vi "RT Main FPGA Test.vi"() -> ()   [LabVIEW 2014]
uses:
  controls/FPGA VI Reference.ctl
  controls/Master Configuration.ctl
  controls/EPICS Configuration.ctl
  Globals/Global - All RT Loop Stop.vi
  Globals/Global - Monitoring Variables.vi
  Globals/Global - Configuration Options.vi
  support/Message Queue/Message Queue.lvlib
  <vilib>/nisyscfg/nisyscfg.lvlib
panel:
  in  "Index":u32
  in  "Message":string
  in  "Send":bool
  in  "stop":bool
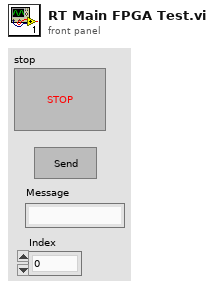
[diagram p1: front panel]
types:
  T1 = typedef "FPGA VI Reference.ctl" = refnum<k20>
  T2 = typedef "Master Configuration.ctl" = cluster{"Thresholds":dbl[], "Epics Configuration":T3, "Epics Configuration File":string, "Number of Channels":dbl}
  T3 = typedef "EPICS Configuration.ctl" = cluster{"Data rate":u32, "Input active":bool[], "# Samples Post Trig":u32, "Armed":bool}
  T4 = typedef "Message Queue.lvlib/All Real-Time Message Queues.ctl" = cluster{"Message Handler":refnum<queue>, "FPGA Subsystem":refnum<queue>}
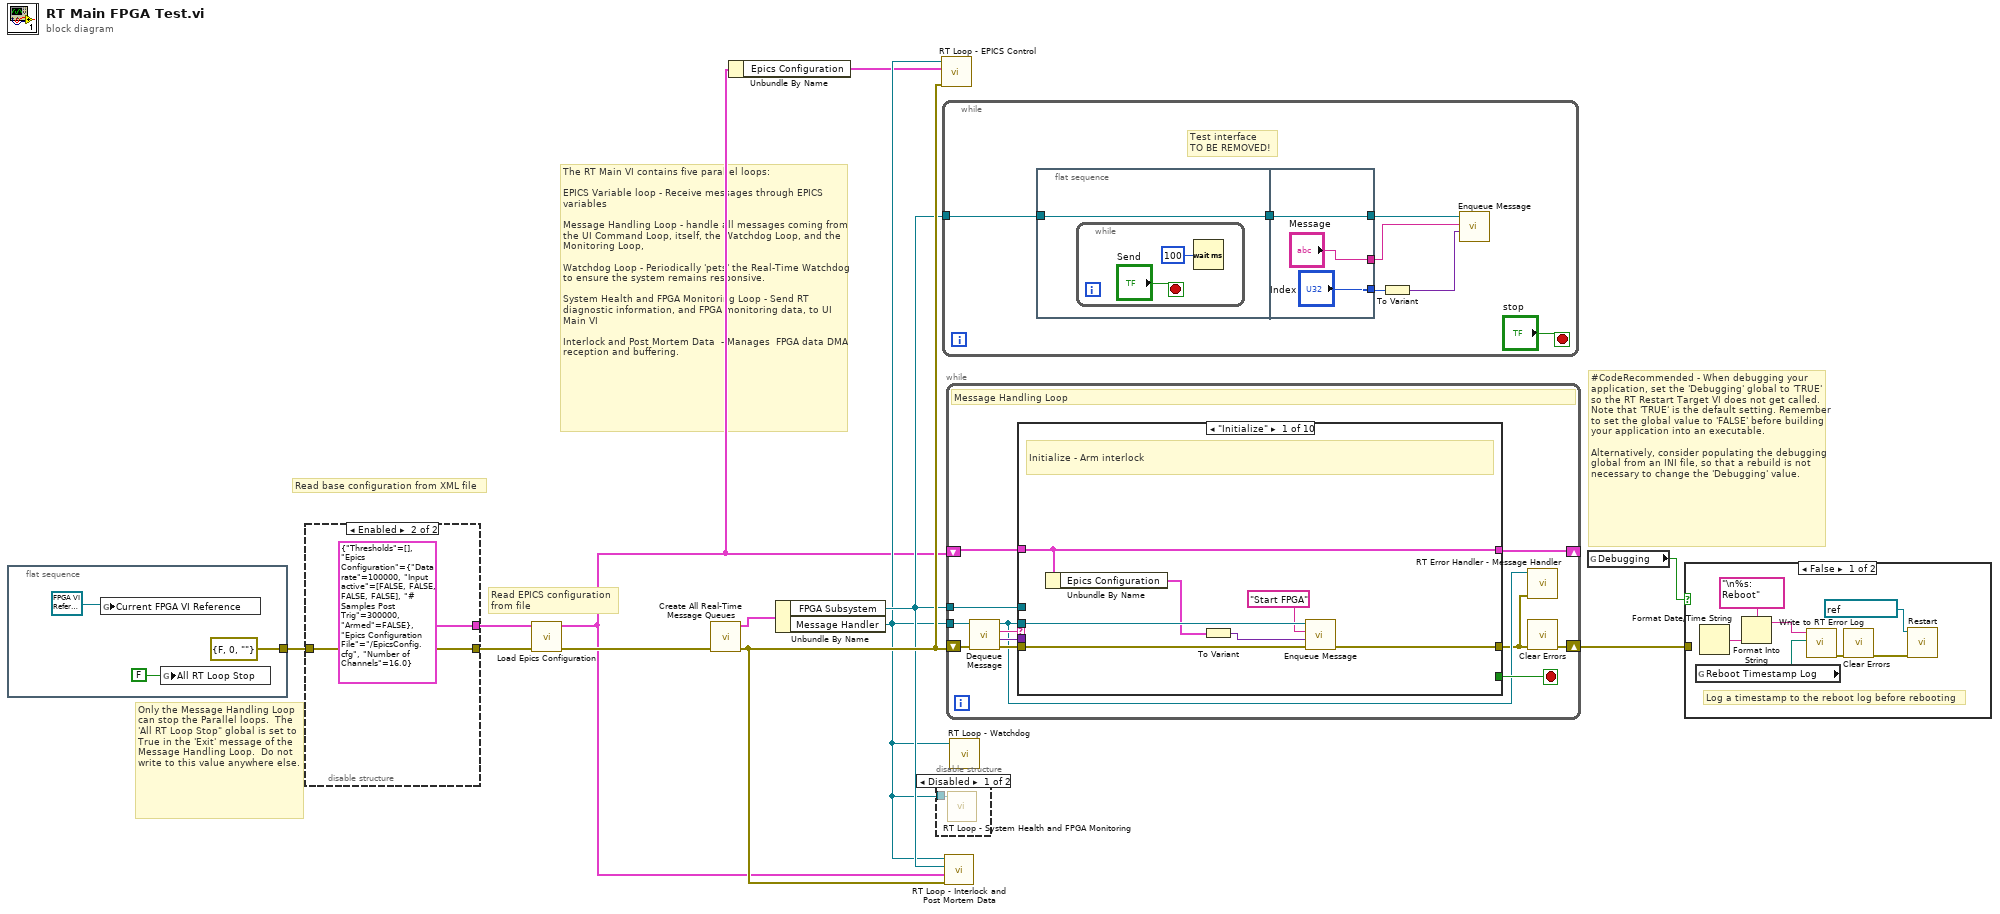
[diagram p0: block diagram]
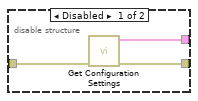
[diagram p3: hidden frame]
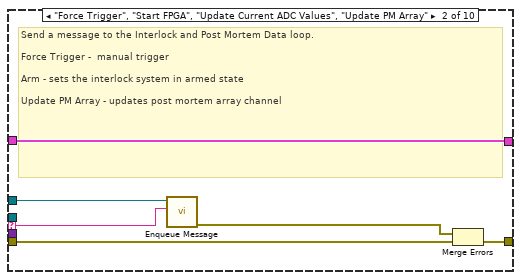
[diagram p5: hidden frame]
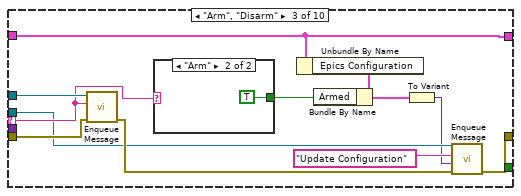
[diagram p6: hidden frame]
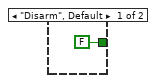
[diagram p7: hidden frame]
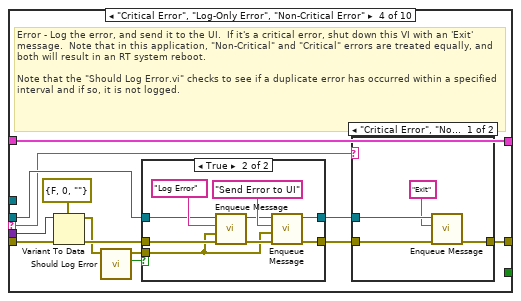
[diagram p8: hidden frame]
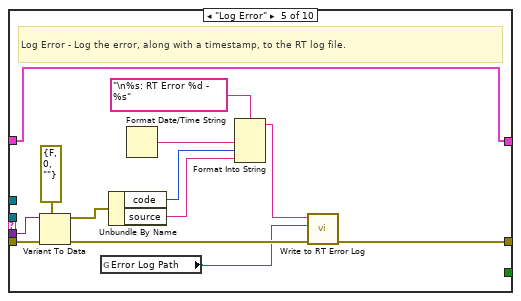
[diagram p11: hidden frame]
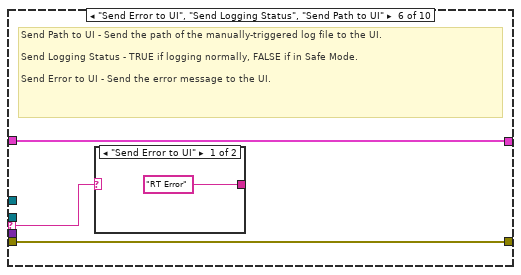
[diagram p12: hidden frame]
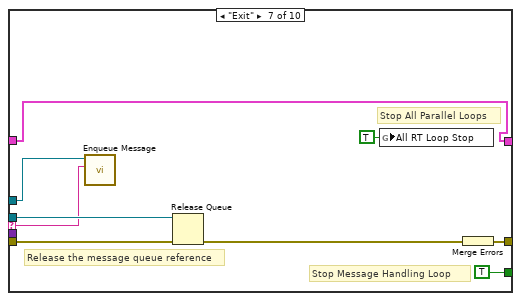
[diagram p14: hidden frame]
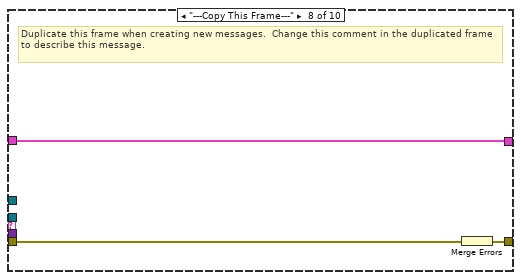
[diagram p15: hidden frame]
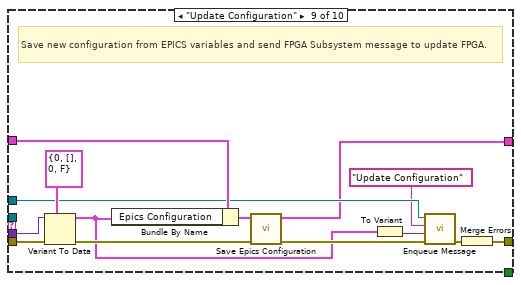
[diagram p16: hidden frame]
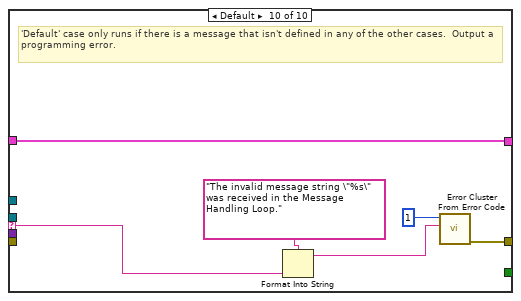
[diagram p17: hidden frame]
diagram:
  # "Read EPICS configuration\nfrom file"
  # "Read base configuration from XML file"
  # "#CodeRecommended - When debugging your application, set the 'Debugging' global to 'TRUE' so the RT Restart Target VI does not get called.  Note that 'TRUE' is the default setting. Remember to set the global value to 'FALSE' before building your application into an executable.\n\nAlternatively, consider populating the debugging global from an INI file, so that a rebuild is not necessary to change the 'Debugging' value."
  # "The RT Main VI contains five parallel loops:\n\nEPICS Variable loop - Receive messages through EPICS variables\n\nMessage Handling Loop - handle all messages coming from the UI Command Loop, itself, the Watchdog Loop, and the Monitoring Loop, \n\nWatchdog Loop - Periodically 'pets' the Real-Time Watchdog to ensure the system remains responsive.\n\nSystem Health and FPGA Monitoring Loop - Send RT diagnostic information, and FPGA monitoring data, to UI Main VI\n\nInterlock and Post Mortem Data  - Manages  FPGA data DMA reception and buffering."
  # "Only the Message Handling Loop can stop the Parallel loops.  The 'All RT Loop Stop\" global is set to True in the 'Exit' message of the Message Handling Loop.  Do not write to this value anywhere else."
  n1 = flat-sequence {
    tunnel: [errorcluster {"status"=FALSE, "code"=0, "source"=""} ("error constant")] -> w12
    frame #0 {
      n2 = global write "Global - Monitoring Variables.vi" "Current FPGA VI Reference"(T1 refnum ("Current FPGA VI Reference")) -> ()
      n3 = global write "Global - All RT Loop Stop.vi" "All RT Loop Stop"(FALSE) -> ()
    }
  }
  n4 = disable-structure shown="Enabled" {
    disable-tunnel: w12 -> [w18 w19]
    disable-tunnel: [w17 w19] -> w6
    disable-tunnel: [w16 T2 {"Thresholds"=[], "Epics Configuration"={"Data rate"=100000, "Input active"=[FALSE, FALSE, FALSE, FALSE], "# Samples Post Trig"=300000, "Armed"=FALSE}, "Epics Configuration File"="/EpicsConfig.cfg", "Number of Channels"=16.0} ("Acquisition and Logging Configuration")] -> w4
    frame Disabled {
      n5 = call "Get Configuration Settings.vi"("error in (no error)"=w18) -> ("error out"=w17:errorcluster, "Acquisition and Logging Configuration"=w16:T2)  [unwired: 9 in]
    }
    frame Enabled {
    }
  }
  n6 = call "Load Epics Configuration.vi"("error in (no error)"=w6, "Master Configuration in"=w4) -> ("error out"=w5:errorcluster, "Master Configuration out"=w2:T2)  [unwired: 8 in]
  n7 = call "Create All Real-Time Message Queues.vi"("error in (no error)"=w5) -> ("error out"=w8:errorcluster, "Message Queues out"=w9:T4)  [unwired: 9 in]
  n8 = Unbundle By Name(w2) -> ("Epics Configuration"=w1:T3)
  n9 = Unbundle By Name(w9) -> ("FPGA Subsystem"=w7:refnum<queue>, "Message Handler"=w3:refnum<queue>)
  n10 = disable-structure shown="Disabled" {
    disable-tunnel: w3 -> [w21 _]
    frame Disabled {
      n11 = call "RT Loop - System Health and FPGA Monitoring.vi"("Message Queue"=w21) -> ()  [unwired: 11 in]
    }
    frame Enabled {
    }
  }
  n12 = call "RT Loop - EPICS Control.vi"("Error"=w8, "Epics Configuration"=w1, "Message Handler"=w3) -> ()  [unwired: 9 in]
  n13 = while {
    tunnel: w7 -> [w27]
    stop <- "stop" stop-if-true
    # "Test interface\nTO BE REMOVED!"
    n14 = flat-sequence {
      tunnel: w27 -> [w29]
      tunnel: [w29] -> w25
      tunnel: [w34] -> w26
      tunnel: w25 -> [w34]
      tunnel: ["Message"] -> w24
      tunnel: ["Index"] -> w23
      frame #0 {
        n15 = while {
          stop <- "Send" stop-if-true
          n16 = Wait (ms)(milliseconds to wait=u32 100) -> ()  [unwired: 1 out]
        }
      }
      frame #1 {
      }
    }
    n17 = To Variant(anything=w23) -> (Variant=w22:variant)
    n18 = call "Enqueue Message.vi"("Message Data"=w22, "Message"=w24, "Message Queue"=w26) -> ()  [unwired: 7 in, 2 out]
  }
  n19 = call "RT Loop - Interlock and Post Mortem Data.vi"("error in (no error)"=w8, "Master Configuration"=w2, "FPGA Subsystem"=w7, "Message Handler"=w3) -> ()  [unwired: 8 in]
  n20 = while {
    tunnel: w3 -> [w41]
    shift-right: [w39] -> w11
    shift-left: w8 -> [w45]
    tunnel: w7 -> [w37]
    shift-right: [w35] -> _
    shift-left: w2 -> [w36]
    stop <- w46 stop-if-true
    # "Message Handling Loop"
    n21 = call "Dequeue Message.vi"("error in (no error)"=w45, "Message Queue"=w41) -> ("error out"=w44:errorcluster, "Message Data"=w42:variant, "Message"=w43:string, "dup Message Queue"=w40:refnum<queue>)  [unwired: 6 in]
    n22 = case "Message Cases" shown="\"Initialize\"" w43 {
      selector: w43 -> [_ w57 w70 w80 _ w117 w122 _ _ w151]
      tunnel: w40 -> [w53 _ w66 w81 _ _ w129 _ _ _]
      tunnel: w44 -> [w52 w59 w68 w83 w115 w118 w125 w132 w146 _]
      tunnel: [w51 w56 w65 w86 w106 w118 w126 w131 w145 w149] -> w38
      tunnel: [_ _ _ _ _ _ TRUE _ _ _] -> w46
      tunnel: w42 -> [_ _ _ w75 w114 _ _ _ w144 _]
      tunnel: w37 -> [_ w58 w71 _ _ _ w123 _ w138 _]
      tunnel: w36 -> [w49 w54 w61 w74 w103 w116 w121 w130 w142 w147]
      tunnel: [w49 w54 w61 w74 w103 w116 w121 w130 w134 w147] -> w35
      frame "Initialize" {
        # "Initialize - Arm interlock"
        n23 = Unbundle By Name(w49) -> ("Epics Configuration"=w48:T3)
        n24 = To Variant(anything=w48) -> (Variant=w47:variant)
        n25 = call "Enqueue Message.vi"("error in (no error)"=w52, "Message Data"=w47, "Message"="Start FPGA", "Message Queue"=w53) -> ("error out"=w51:errorcluster)  [unwired: 6 in, 1 out]
      }
      frame "Force Trigger", "Start FPGA", "Update Current ADC Values", "Update PM Array" {
        # "Send a message to the Interlock and Post Mortem Data loop.\n\nForce Trigger -  manual trigger\n\nArm - sets the interlock system in armed state\n\nUpdate PM Array - updates post mortem array channel"
        n26 = call "Enqueue Message.vi"("Message"=w57, "Message Queue"=w58) -> ("error out"=w55:errorcluster)  [unwired: 8 in, 1 out]
        n27 = Merge Errors(w55, w59) -> (w56:errorcluster)
      }
      frame "Arm", "Disarm" {
        n28 = call "Enqueue Message.vi"("error in (no error)"=w68, "Message"=w70, "Message Queue"=w71) -> ("error out"=w67:errorcluster)  [unwired: 7 in, 1 out]
        n29 = case shown="\"Arm\"" w70 {
          tunnel: [FALSE ("Armed") TRUE ("Armed")] -> w69
          frame "Disarm", Default {
          }
          frame "Arm" {
          }
        }
        n30 = Unbundle By Name(w61) -> ("Epics Configuration"=w60:T3)
        n31 = Bundle By Name(cluster=w60, "Armed"=w69) -> (w63:T3)
        n32 = To Variant(anything=w63) -> (Variant=w62:variant)
        n33 = call "Enqueue Message.vi"("error in (no error)"=w67, "Message Data"=w62, "Message"="Update Configuration", "Message Queue"=w66) -> ("error out"=w65:errorcluster)  [unwired: 6 in, 1 out]
      }
      frame "Critical Error", "Log-Only Error", "Non-Critical Error" {
        # "Error - Log the error, and send it to the UI.  If it's a critical error, shut down this VI with an 'Exit' message.  Note that in this application, \"Non-Critical\" and \"Critical\" errors are treated equally, and both will result in an RT system reboot.\n\nNote that the \"Should Log Error.vi\" checks to see if a duplicate error has occurred within a specified interval and if so, it is not logged."
        n34 = Variant To Data(error in=w83, type=errorcluster {"status"=FALSE, "code"=0, "source"=""} ("error out"), Variant=w75) -> (data=w78:errorcluster, error out=w84:errorcluster)
        n35 = call "Should Log Error.vi"("error to report"=w78) -> ("Should Log Error?"=w76:bool, "dup error to report"=w77:errorcluster)  [unwired: 9 in]
        n36 = case shown="True" w76 {
          tunnel: [w88 w95] -> w82
          tunnel: [w87 w94] -> w79
          tunnel: w81 -> [w87 w93]
          tunnel: w84 -> [w88 w90]
          tunnel: w77 -> [_ w89]
          frame False {
          }
          frame True {
            n37 = call "Enqueue Message.vi"("error in (no error)"=w90, "Message Data"=w89, "Message"="Log Error", "Message Queue"=w93) -> ("error out"=w91:errorcluster, "dup Message Queue"=w92:refnum<queue>)  [unwired: 6 in]
            n38 = call "Enqueue Message.vi"("error in (no error)"=w91, "Message Data"=w89, "Message"="Send Error to UI", "Message Queue"=w92) -> ("error out"=w95:errorcluster, "dup Message Queue"=w94:refnum<queue>)  [unwired: 6 in]
          }
        }
        n39 = case shown="\"Critical Error\", \"Non-Critical Error\"" w80 {
          tunnel: w82 -> [w101 w102]
          tunnel: w79 -> [w99 _]
          tunnel: [w100 w102] -> w86
          frame "Critical Error", "Non-Critical Error" {
            n40 = call "Enqueue Message.vi"("error in (no error)"=w101, "Message"="Exit", "Message Queue"=w99) -> ("error out"=w100:errorcluster)  [unwired: 7 in, 1 out]
          }
          frame Default {
          }
        }
      }
      frame "Log Error" {
        # "Log Error - Log the error, along with a timestamp, to the RT log file."
        n41 = Variant To Data(error in=w115, type=errorcluster {"status"=FALSE, "code"=0, "source"=""} ("error constant"), Variant=w114) -> (data=w109:errorcluster, error out=w112:errorcluster)
        n42 = global read "Global - Configuration Options.vi" "Error Log Path"() -> (w104:path)
        n43 = Unbundle By Name(w109) -> ("code"=w108:i32, "source"=w107:string)
        n44 = Format Date/Time String() -> (date/time string=w110:string)  [unwired: 3 in]
        n45 = Format Into String(format string="\n%s: RT Error %d - %s", w110, w108, w107) -> (resulting string=w105:string)  [unwired: 2 in, 1 out]
        n46 = call "Write to RT Error Log.vi"("error in (no error)"=w112, "Error Log Path"=w104, "Log Entry"=w105) -> ("error out"=w106:errorcluster)  [unwired: 8 in]
      }
      frame "Send Error to UI", "Send Logging Status", "Send Path to UI" {
        # "Send Path to UI - Send the path of the manually-triggered log file to the UI.\n\nSend Logging Status - TRUE if logging normally, FALSE if in Safe Mode.\n\nSend Error to UI - Send the error message to the UI."
        n47 = case shown="\"Send Error to UI\"" w117 {
          selector: w117 -> [_ w120]
          tunnel: ["RT Error" ("Message") w120] -> _
          frame "Send Error to UI" {
          }
          frame Default {
          }
        }
      }
      frame "Exit" {
        # "Stop Message Handling Loop"
        # "Stop All Parallel Loops"
        # "Release the message queue reference"
        n48 = call "Enqueue Message.vi"("Message"=w122, "Message Queue"=w123) -> ()  [unwired: 8 in, 2 out]
        n49 = Release Queue(queue=w129, error in (no error)=w125) -> (error out=w127:errorcluster)  [unwired: 1 in, 2 out]
        n50 = global write "Global - All RT Loop Stop.vi" "All RT Loop Stop"(TRUE ("Stop Monitoring Loops")) -> ()
        n51 = Merge Errors(w127) -> (w126:errorcluster)
      }
      frame "---Copy This Frame---" {
        # "Duplicate this frame when creating new messages.  Change this comment in the duplicated frame to describe this message."
        n52 = Merge Errors(w132) -> (w131:errorcluster)
      }
      frame "Update Configuration" {
        # "Save new configuration from EPICS variables and send FPGA Subsystem message to update FPGA."
        n53 = Variant To Data(error in=w146, type=T3 {"Data rate"=0, "Input active"=[], "# Samples Post Trig"=0, "Armed"=FALSE} ("Epics Configuration"), Variant=w144) -> (data=w133:T3, error out=w141:errorcluster)
        n54 = Bundle By Name(cluster=w142, "Epics Configuration"=w133) -> (w135:T2)
        n55 = call "Save Epics Configuration.vi"("error in (no error)"=w141, "Master Configuration in"=w135) -> ("error out"=w136:errorcluster, "Master Configuration out"=w134:T2)  [unwired: 8 in]
        n56 = To Variant(anything=w133) -> (Variant=w139:variant)
        n57 = call "Enqueue Message.vi"("error in (no error)"=w136, "Message Data"=w139, "Message"="Update Configuration", "Message Queue"=w138) -> ("error out"=w140:errorcluster)  [unwired: 6 in, 1 out]
        n58 = Merge Errors(w140) -> (w145:errorcluster)
      }
      frame Default {
        # "'Default' case only runs if there is a message that isn't defined in any of the other cases.  Output a programming error."
        n59 = Format Into String(format string="The invalid message string \"%s\" was received in the Message Handling Loop." ("Unknown Message Error Text"), w151) -> (resulting string=w148:string)  [unwired: 2 in, 1 out]
        n60 = call <vilib>:"Error Cluster From Error Code.vi"("error message (\"\")"=w148, "error code (0)"=1) -> ("error out"=w149:errorcluster)  [unwired: 7 in]
      }
    }
    n61 = call "RT Error Handler - Message Handler.vi"("error in (no error)"=w38, "Message Queue"=w40) -> ()  [unwired: 9 in, 1 out]
    n62 = call <vilib>:"Clear Errors.vi"("error in (no error)"=w38) -> ("error out"=w39:errorcluster)  [unwired: 5 in, 1 out]
  }
  n63 = call "RT Loop - Watchdog.vi"("Message Queue"=w3) -> ()  [unwired: 11 in]
  n64 = global read "Global - Configuration Options.vi" "Debugging"() -> (w10:bool)
  n65 = case shown="False" w10 {
    tunnel: w11 -> [_ _]
    frame False {
      # "Log a timestamp to the reboot log before rebooting"
      n66 = global read "Global - Configuration Options.vi" "Reboot Timestamp Log"() -> (w155:path)
      n67 = Format Date/Time String() -> (date/time string=w157:string)  [unwired: 3 in]
      n68 = Format Into String(format string="\n%s: Reboot", w157) -> (resulting string=w156:string)  [unwired: 2 in, 1 out]
      n69 = call "Write to RT Error Log.vi"("Error Log Path"=w155, "Log Entry"=w156) -> ("error out"=w159:errorcluster)  [unwired: 9 in]
      n70 = call <vilib>:"Clear Errors.vi"("error in (no error)"=w159) -> ("error out"=w154:errorcluster)  [unwired: 5 in, 1 out]
      n71 = call <vilib>:"Restart.vi"("error in (no error)"=w154, "Session in"=refnum<k21> "localhost" ("session in")) -> ()  [unwired: 7 in, 3 out]
    }
    frame True {
    }
  }
